vi "Return Value Manifester VI Path.vi"(11 "Identity Writer in":refnum<class "Identity Writer.lvclass">) -> (2 "Manifester VI Path":path, 3 "Identity Writer out":refnum<class "Identity Writer.lvclass">)   [LabVIEW 2013, in "Identity Writer.lvclass"]
uses:
  Identity Writer.lvclass
  Manifestation Writer/Manifestation Writer.lvclass/Manifestation Writer.ctl
  Manifestation Writer/Manifestation Writer.lvclass
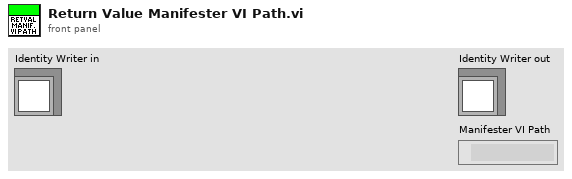
[diagram p1: front panel]
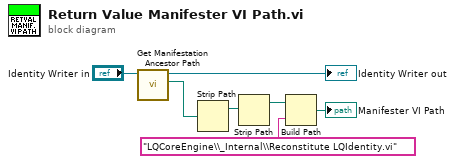
[diagram p0: block diagram]
diagram:
  n1 = call "Get Manifestation Ancestor Path.vi"("Manifestation Writer in"="Identity Writer in") -> ("Manifestation Ancestor Path"=w3:path, "Manifestation Writer out"=→"Identity Writer out":refnum<class "Identity Writer.lvclass">)  [unwired: 9 in]
  n2 = Strip Path(path=w3) -> (stripped path=w7:path)  [unwired: 1 out]
  n3 = Strip Path(path=w7) -> (stripped path=w6:path)  [unwired: 1 out]
  n4 = Build Path(base path=w6, name or relative path="LQCoreEngine\\_Internal\\Reconstitute LQIdentity.vi") -> (appended path=→"Manifester VI Path":path)
